vi "Apply DevInfo.vi"(8 "error in (no error)":errorcluster, 10 "DevInfo":refnum<class "DevInfo.lvclass">, 11 "Hardware in":refnum<class "Hardware.lvclass">) -> (0 "error out":errorcluster, 3 "Hardware out":refnum<class "Hardware.lvclass">)   [LabVIEW 2016, in "Hardware.lvlib" / "Hardware.lvclass"]
uses:
  <userlib>/Common Components/Hardware/Abstract Hardware/Hardware.lvclass
  <userlib>/Common Components/Hardware/DevInfo/DevInfo.lvclass
  <userlib>/Common Components/Hardware/DevInfo/DevInfo.lvclass/DevInfo.ctl
  <userlib>/Common Components/Hardware/Abstract Hardware/Hardware.lvclass/Hardware.ctl
  <userlib>/Common Components/Hardware/DevInfo/Read Device Name.vi
  <userlib>/Common Components/Hardware/DevInfo/Read Label.vi
  <userlib>/Common Components/Hardware/DevInfo/Read GUID.vi
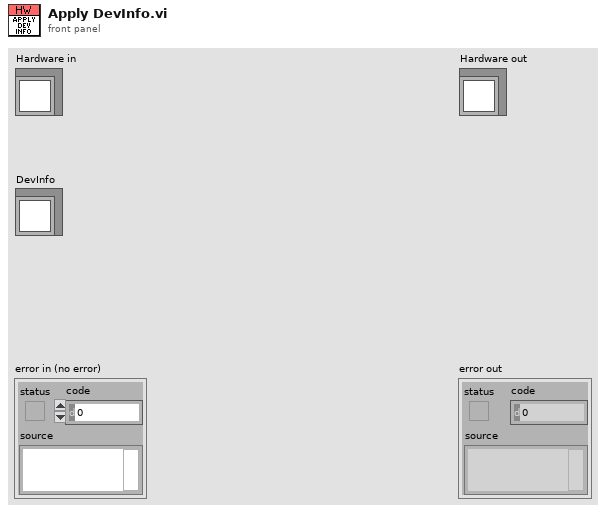
[diagram p1: front panel]
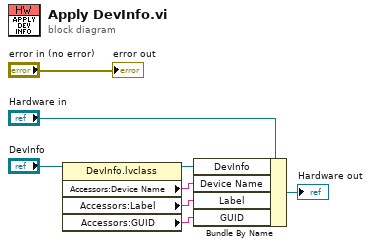
[diagram p0: block diagram]
diagram:
  n1 = property class="DevInfo.lvclass"(reference="DevInfo") -> (reference out=w4:refnum<class "DevInfo.lvclass">, "Accessors:Device Name"=w3:string, "Accessors:Label"=w2:string, "Accessors:GUID"=w1:string)  [unwired: 1 in, 1 out]
  n2 = Bundle By Name(cluster="Hardware in", "DevInfo"=w4, "Device Name"=w3, "Label"=w2, "GUID"=w1) -> (→"Hardware out":refnum<class "Hardware.lvclass">)
  "error out" <- "error in (no error)"
